vi "Create Instance Impl.vi"(8 "error in (no error)":errorcluster, 10 "Stage Configuration":T1={"Serial Port"="COM4", "Forward Step (mm)"=0.4, "Lane Length (mm)"=6.0, "Lane Separation (mm)"=0.8, "Stage Type"=enum."Ti2", "Autofocus Z Planes"=9, "Autofocus Range (um)"=30.0, "Stage Limits"={"Y Min"=-4.5, "Y Max"=3.0, "X Min"=-19.0, "X Max"=33.5}, "Slide (mm)"={"top"=-13.0, "right"=-22.3, "width"=60.0, "height"=25.4}}, 11 "Simulated Stage in":refnum<class "Simulated Stage.lvclass">) -> (0 "error out":errorcluster, 3 "Simulated Stage out":refnum<class "Simulated Stage.lvclass">)   [LabVIEW 2023, in "Simulated Stage.lvlib" / "Simulated Stage.lvclass"]
uses:
  Resources/Type Defs/Stage Configuration.ctl
  Simulated Stage.lvclass
  Simulated Stage.lvclass/Simulated Stage.ctl
  Resources/Type Defs/Stage Position.ctl
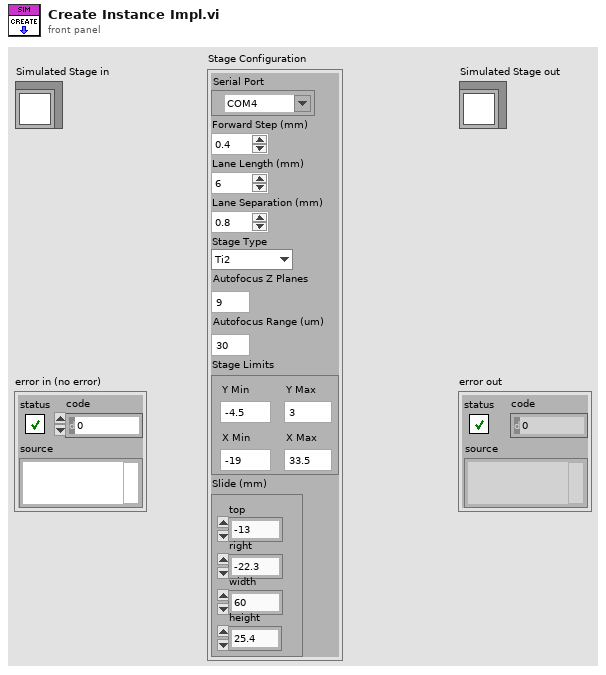
[diagram p1: front panel]
types:
  T1 = typedef "Stage Configuration.ctl" = cluster{"Serial Port":refnum<visa-resource-name>, "Forward Step (mm)":dbl, "Lane Length (mm)":dbl, "Lane Separation (mm)":dbl, "Stage Type":enum16{"Disabled", "ESP301", "Ti2", "Ludl", "ASI", "Simulate"}, "Autofocus Z Planes":i32, "Autofocus Range (um)":dbl, "Stage Limits":cluster{"Y Min":dbl, "Y Max":dbl, "X Min":dbl, "X Max":dbl}, "Slide (mm)":cluster{"top":dbl, "right":dbl, "width":dbl, "height":dbl}}
  T2 = typedef "Stage Position.ctl" = cluster{"X (mm)":dbl, "Y (mm)":dbl, "Z (mm)":dbl}
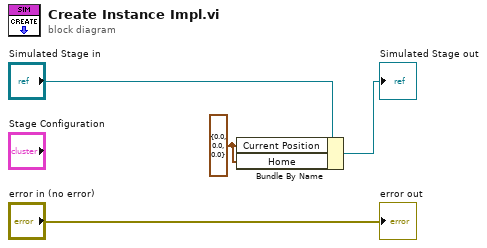
[diagram p0: block diagram]
diagram:
  w1 = T2 {"X (mm)"=0.0, "Y (mm)"=0.0, "Z (mm)"=0.0} ("Current Position")
  n1 = Bundle By Name(cluster="Simulated Stage in", "Current Position"=w1, "Home"=w1) -> (→"Simulated Stage out":refnum<class "Simulated Stage.lvclass">)
  "error out" <- "error in (no error)"
